vi "rec_solutionChangeDAQreplicates_v02.vi"(0 "AI task in":refnum<k21>, 1 "number of samples":i32=-1, 2 "controls array in":refnum<vi>[](array[refnum]), 3 "daq_do":tag="Dev1/ai0:1", 4 "AO task in":refnum<k21>, 5 "error in":errorcluster, 6 "Start Position":T1(ring), 7 "Jump On Time (s)":dbl, 9 "Duration (s)":dbl, 10 "Jump Position":T1(ring), 11 "Jump Duration (s)":dbl, 12 "common cluster":T2) -> (14 "AI task out":refnum<k21>, 15 "data out (pA or mV)":waveform(dbl)(graph), 16 "control array out":refnum<vi>[](array[refnum]), 18 "AO task out":refnum<k21>, 19 "error out":errorcluster)   [LabVIEW 2019]
uses:
  multipatch/controls/multipatch_common_controls_v4.ctl
  machine_vision/controls/transform_cluster_actuator.ctl
  machine_vision/coordinate model vis/transform_properties_actuators.ctl
  pipette cleaning/pressure box/cleaning_soft/controls/actuator_cluster.ctl
  pipette cleaning/pressure box/cleaning_soft/controls/actuator_type.ctl
  pipette cleaning/pressure box/cleaning_soft/controls/pressure_box_control.ctl
  pipette cleaning/pressure box/cleaning_soft/controls/pressure_box_type.ctl
  controls/NH_method.ctl
  <vilib>/DAQmx/read.llb/DAQmx Read (Analog Wfm 1Chan NSamp).vi
  <vilib>/DAQmx/miscellaneous.llb/DAQmx Fill In Error Info.vi
  <resource>/objmgr/daqmx.rc
panel:
  out "AvailSampPerChan":u32
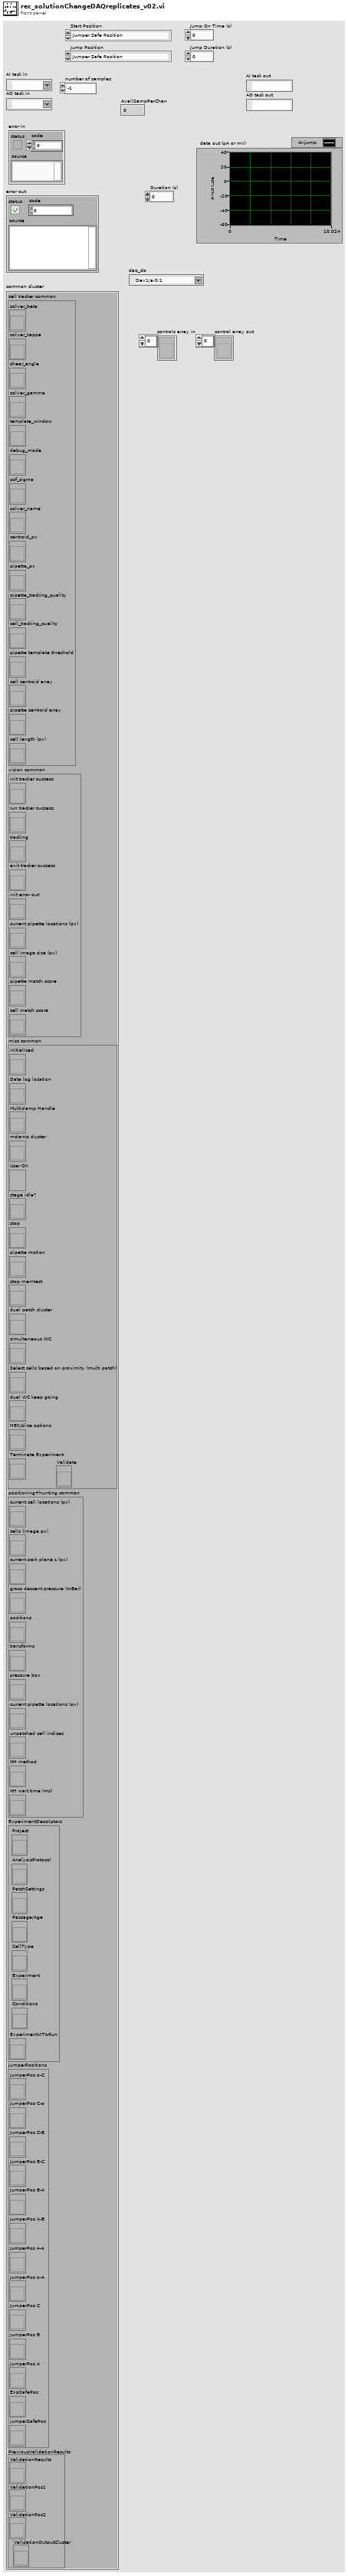
[diagram p1: front panel]
types:
  T1 = enum16{"Jumper Safe Position", "Experiment Safe Position", "Jumper Position A", "Jumper Position B", "Jumper Position C", "Jumper Position o-A", "Jumper Position A-o", "Jumper Position A-B", "Jumper Position B-A", "Jumper Position B-C", "Jumper Position C-B", "Jumper Position C-o", "Jumper Position o-C"}
  T2 = typedef "multipatch_common_controls_v4.ctl" = cluster{"cell tracker common":cluster{"solver_beta":refnum<vi>, "solver_kappa":refnum<vi>, "shear_angle":refnum<vi>, "solver_gamma":refnum<vi>, "template_window":refnum<vi>, "debug_mode":refnum<vi>, "psf_sigma":refnum<vi>, "solver_name":refnum<vi>, "centroid_px":refnum<vi>, "pipette_px":refnum<vi>, "pipette_tracking_quality":refnum<vi>, "cell_tracking_quality":refnum<vi>, "pipette template threshold":refnum<vi>, "cell centroid array":refnum<vi>, "pipette centroid array":refnum<vi>, "cell length (px)":refnum<vi>}, "vision common":cluster{"init tracker success":refnum<vi>, "run tracker success":refnum<vi>, "tracking":refnum<vi>, "exit tracker success":refnum<vi>, "init error out":refnum<vi>, "current pipette locations (px)":refnum<vi>, "cell image size (px)":refnum<vi>, "pipette match score":refnum<vi>, "cell match score":refnum<vi>}, "misc common":cluster{"initialized":refnum<vi>, "Data log location":refnum<vi>, "Multiclamp Handle":refnum<vi>, "mclamp cluster":refnum<vi>, "User OK":refnum<vi>, "stage idle?":refnum<vi>, "stop":refnum<vi>, "pipette motion":refnum<vi>, "stop memtest":refnum<vi>, "dual patch cluster":refnum<vi>, "simultaneous WC":refnum<vi>, "Select cells based on proximity (multi patch)":refnum<vi>, "dual WC keep going":refnum<vi>, "HEK/slice options":refnum<vi>, "Terminate Experiment":refnum<vi>, "Validate":refnum<vi>}, "positioning+hunting common":cluster{"current cell locations (px)":refnum<vi>, "cells (image px)":refnum<vi>, "current park plane z (px)":refnum<vi>, "gross descent pressure (mBar)":refnum<vi>, "positions":refnum<vi>, "transforms":refnum<vi>, "pressure box":refnum<vi>, "current pipette locations (px)":refnum<vi>, "unpatched cell indices":refnum<vi>, "NH method":refnum<vi>, "NH wait time (ms)":refnum<vi>}, "ExperimentDescriptors":cluster{"Project":refnum<vi>, "AnalysisProtocol":refnum<vi>, "PatchSettings":refnum<vi>, "Passage/Age":refnum<vi>, "CellType":refnum<vi>, "Experiment":refnum<vi>, "Conditions":refnum<vi>, "ExperimentVIToRun":refnum<vi>}, "JumperPositions":cluster{"JumperPos o-C":refnum<vi>, "JumperPos C-o":refnum<vi>, "JumperPos C-B":refnum<vi>, "JumperPos B-C":refnum<vi>, "JumperPos B-A":refnum<vi>, "JumperPos A-B":refnum<vi>, "JumperPos A-o":refnum<vi>, "JumperPos o-A":refnum<vi>, "JumperPos C":refnum<vi>, "JumperPos B":refnum<vi>, "JumperPos A":refnum<vi>, "ExpSafePos":refnum<vi>, "jumperSafePos":refnum<vi>}, "PreviousValidationResults":cluster{"ValidationResults":refnum<vi>, "ValidationPos1":refnum<vi>, "ValidationPos2":refnum<vi>, "ValidationOutputCluster":refnum<vi>}}
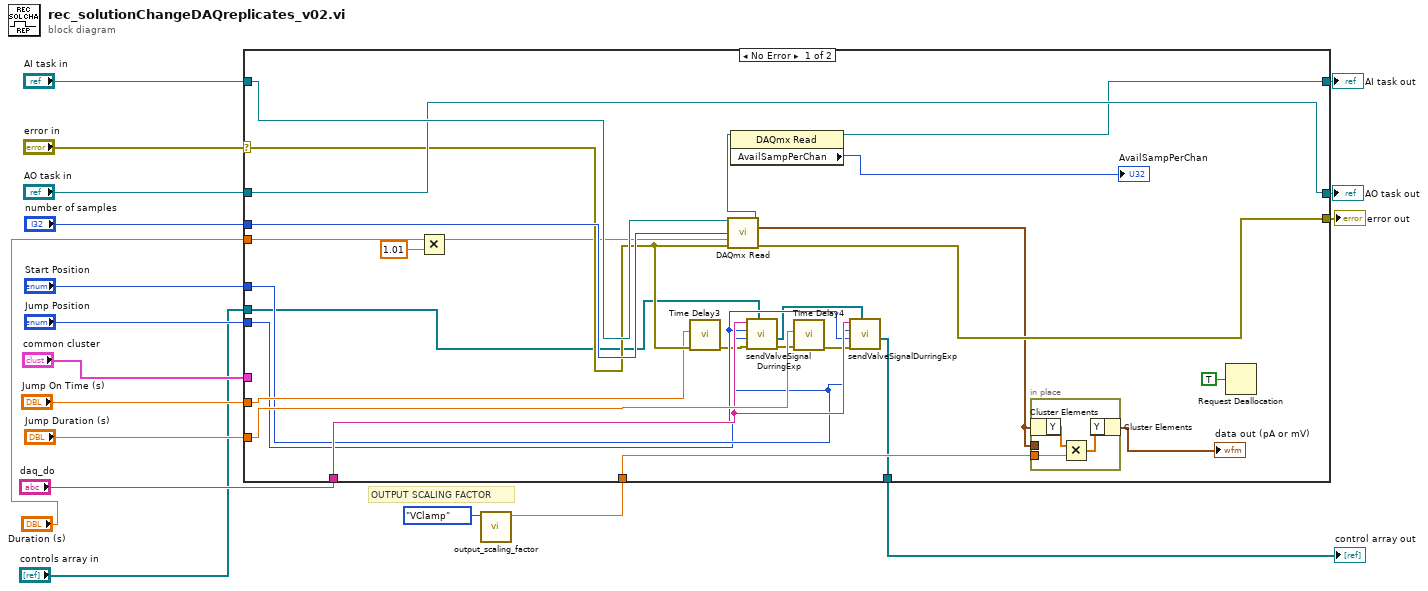
[diagram p0: block diagram]
diagram:
  # "OUTPUT SCALING FACTOR"
  n1 = call "output_scaling_factor.vi"("which clamp"=enum16{"VClamp", "IClamp"}."VClamp") -> ("output scaling factor"=w12:dbl)  [unwired: 10 in]
  n2 = case shown="No Error" "error in" {
    selector: "error in" -> [w39 w49]
    tunnel: "AI task in" -> [w43 w51]
    tunnel: "AO task in" -> [w41 w50]
    tunnel: [w41 w50] -> w15
    tunnel: [w31 w51] -> w14
    tunnel: [w42 w49] -> w13
    tunnel: w12 -> [w44 _]
    tunnel: "number of samples" -> [w40 _]
    tunnel: "common cluster" -> [_ _]
    tunnel: "Jump On Time (s)" -> [w38 _]
    tunnel: "Jump Duration (s)" -> [w37 _]
    tunnel: "Start Position" -> [w35 _]
    tunnel: "Jump Position" -> [w34 _]
    tunnel: "daq_do" -> [w36 _]
    tunnel: "controls array in" -> [w33 w48]
    tunnel: [w32 w48] -> w2
    tunnel: "Duration (s)" -> [w29 _]
    frame No Error {
      n3 = Multiply(x=w29, y=1.01) -> (x*y=w28:dbl)
      n4 = call "Time Delay3"("error in (no error)"=w39, "Delay Time (s)"=w38) -> ("error out"=w24:errorcluster)  [unwired: 9 in]
      n5 = call-poly <vilib>:"DAQmx Read.vi"("task/channels in"=w43, "number of samples per channel"=w40, "timeout"=w28, "error in"=w39) -> ("task out"=w20:refnum<k21>, "data"=w25:waveform(dbl), "error out"=w42:errorcluster)  [unwired: 9 in]
      n6 = property class="DAQmx Read"(reference=w20) -> (reference out=w31:refnum<k21>, "AvailSampPerChan"=→"AvailSampPerChan":u32)  [unwired: 1 in, 1 out]
      n7 = call "sendValveSignalDurringExp.vi"("daq_do"=w36, "ChangeToValve"=w34, "CurrentValve"=w35, "error in"=w24, "controls array in"=w33) -> ("control array out"=w21:refnum<vi>[], "error out"=w23:errorcluster)  [unwired: 3 in, 1 out]
      n8 = call "Time Delay4"("error in (no error)"=w23, "Delay Time (s)"=w37) -> ("error out"=w22:errorcluster)  [unwired: 9 in]
      n9 = call "sendValveSignalDurringExp.vi"("daq_do"=w36, "ChangeToValve"=w35, "CurrentValve"=w34, "error in"=w22, "controls array in"=w21) -> ("control array out"=w32:refnum<vi>[])  [unwired: 3 in, 2 out]
      n10 = in-place {
        in-place-border: w44 -> [w47]
        in-place-border: w25 -> [_]
        n11 = in-place-cluster #1(w25) -> ("Y"=w46:dbl[])
        n12 = Multiply(x=w46, y=w47) -> (x*y=w45:dbl[])
        n13 = in-place-cluster #1("Y"=w45) -> (→"data out (pA or mV)":waveform(dbl))
      }
      n14 = Request Deallocation(TRUE ("flag")) -> ()
    }
    frame Error {
    }
  }
  "AI task out" <- w14
  "AO task out" <- w15
  "error out" <- w13
  "control array out" <- w2
